vi "GetText.vi"(8 "error in":errorcluster, 11 "node in":refnum<class "ActionVI.lvclass">) -> (0 "error out":errorcluster, 1 "additional text":string, 2 "text":string, 3 "node out":refnum<class "ActionVI.lvclass">, 4 "glyph":string)   [LabVIEW 2015, in "ActionVI.lvclass"]
doc: "Returns the text representation of the node used for the tree control."
uses:
  ActionVI.lvclass
  ActionVI.lvclass/ActionVI.ctl
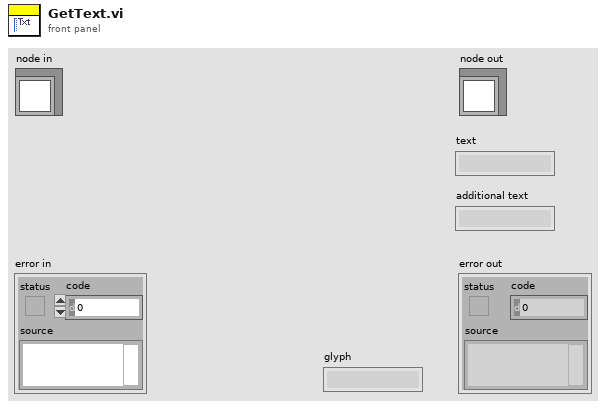
[diagram p1: front panel]
types:
  T1 = typedef "ActionVITypes.ctl" = enum16{"OnDelete", "OnLoad", "OnSystemShutdown", "OnSave", "OnDownload", "OnPaste", "OnTargetTypeChange", "OnDeleteRequest", "OnCompile"}
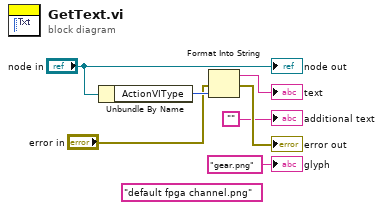
[diagram p0: block diagram]
diagram:
  (unwired) "default fpga channel.png" ("glyph")
  n1 = Unbundle By Name("node in") -> ("ActionVIType"=w6:T1)
  n2 = Format Into String(error in="error in", w6) -> (resulting string=→"text":string, error out=→"error out":errorcluster)  [unwired: 2 in]
  "node out" <- "node in"
  "additional text" <- ""
  "glyph" <- "gear.png" ("glyph")
